vi "CaptParameters.vi"() -> ()   [LabVIEW 2012]
panel:
  in  "CaptParameters":T1={"baudrate"=9600, "databits"=8, "paritybit"=0, "stopbits"=1, "flux control"=0, "Port"="COM1", "Register Address"=17, "Serial Parameters"={"Mode"=enum."RTU", "Slave Address"=1}, "Timeout"=0, "PressureLimit"=0.0}
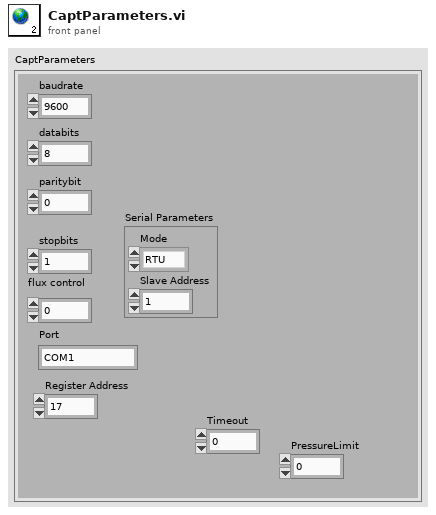
[diagram p1: front panel]
types:
  T1 = cluster{"baudrate":u32, "databits":u16, "paritybit":u16, "stopbits":u16, "flux control":u16, "Port":string, "Register Address":u16, "Serial Parameters":cluster{"Mode":enum16{"RTU", "ASCII"}, "Slave Address":u8}, "Timeout":u32, "PressureLimit":dbl}
diagram:
